vi "draw_menu.vi"(11 "input":picture) -> (3 "menu":picture)   [LabVIEW 2025]
uses:
  <vilib>/Utility/miscctls.llb/LVBoundsTypeDef.ctl
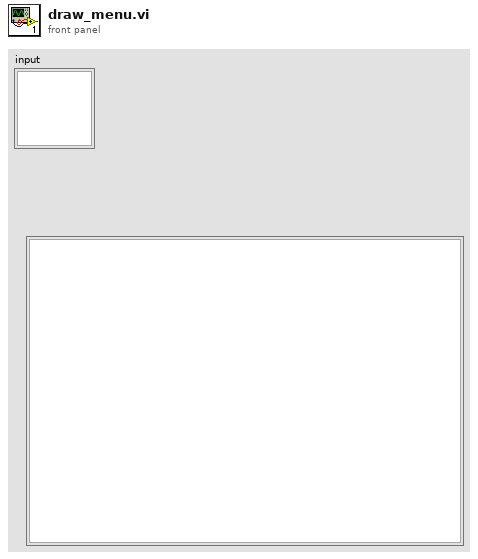
[diagram p1: front panel]
types:
  T1 = cluster{"horizontal":enum16{"left", "center", "right"}, "vertical":enum16{"top", "center", "bottom"}}
  T2 = typedef "LVBoundsTypeDef.ctl" = cluster{"Width":u32, "Height":u32}
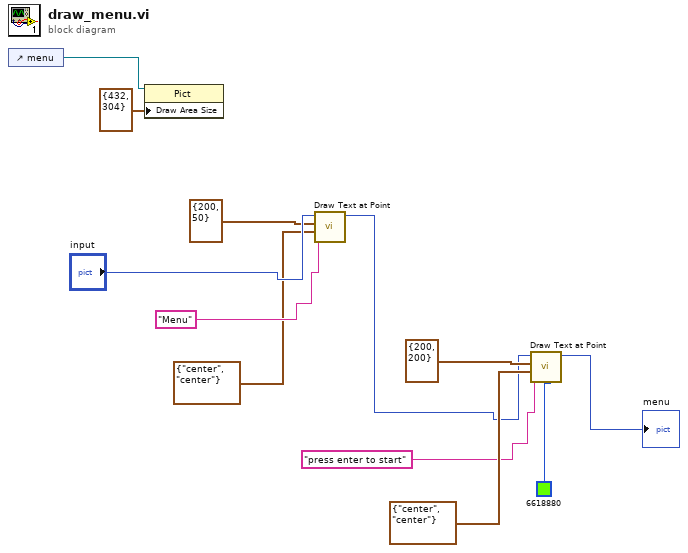
[diagram p0: block diagram]
diagram:
  n1 = control-ref of="menu"() -> (w11:refnum<vi>)
  n2 = property on="Property Node" class="Pict"(reference=w11, "Draw Area Size"=T2 {"Width"=432, "Height"=304}) -> ()  [unwired: 1 in, 2 out]
  n3 = call <vilib>:"Draw Text at Point.vi"("text"="Menu", "alignment(left, top)"=T1 {"horizontal"=enum."center", "vertical"=enum."center"}, "origin"=cluster{"x":i16, "y":i16} {"x"=200, "y"=50}, "picture"="input") -> ("new picture"=w3:picture)  [unwired: 6 in, 1 out]
  n4 = call <vilib>:"Draw Text at Point.vi"("BG color(transparent)"=u32 6618880, "text"="press enter to start", "alignment(left, top)"=T1 {"horizontal"=enum."center", "vertical"=enum."center"}, "origin"=cluster{"x":i16, "y":i16} {"x"=200, "y"=200}, "picture"=w3) -> ("new picture"=→"menu":picture)  [unwired: 5 in, 1 out]
